vi "Register gRPC Methods.vi"(8 "error in (no error)":errorcluster, 11 "Template Server in":refnum<class "MeasurementService_Template.lvclass">) -> (0 "error out":errorcluster, 3 "Template Server out":refnum<class "MeasurementService_Template.lvclass">)   [LabVIEW 2020, in "LoadRegulation.lvlib" / "MeasurementService_Template.lvclass"]
uses:
  MeasurementService_Template.lvclass
  typeDefs/Server Internal UEs.ctl
  typeDefs/Server Internal Message.ctl
  typeDefs/Server gRPC UEs.ctl
  <vilib>/gRPC/LabVIEW gRPC Library/Server API/typeDefs/gRPCId Cluster.ctl
  <vilib>/gRPC/LabVIEW gRPC Library/Server API/typeDefs/grpcId.ctl
  MeasurementService_Template.lvclass/MeasurementService_Template.ctl
  <vilib>/gRPC/LabVIEW gRPC Library/gprc-lvsupport-release.lvlib
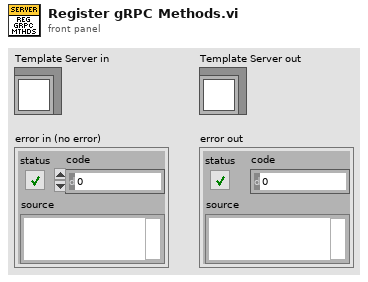
[diagram p1: front panel]
types:
  T1 = typedef "LoadRegulation.lvlib/MeasurementService_Template.lvclass/Server gRPC UEs.ctl" = cluster{"Measurement_v1_MeasurementService_GetMetadata gRPC UE":refnum<user-event>, "Measurement_v1_MeasurementService_Measure gRPC UE":refnum<user-event>, "Measurement_v1_MeasurementService_StopService gRPC UE":refnum<user-event>}
  T2 = typedef "LoadRegulation.lvlib/MeasurementService_Template.lvclass/Server Internal UEs.ctl" = cluster{"Measurement_v1_MeasurementService_GetMetadata Internal UE":refnum<user-event>, "Measurement_v1_MeasurementService_Measure Internal UE":refnum<user-event>, "Measurement_v1_MeasurementService_StopService Internal UE":refnum<user-event>}
  T3 = typedef "gprc-lvsupport-release.lvlib/grpcId.ctl" = u64
  T4 = typedef "LoadRegulation.lvlib/MeasurementService_Template.lvclass/Server Internal Message UE.ctl" = refnum<user-event>
  T5 = typedef "gprc-lvsupport-release.lvlib/gRPCId Cluster UE.ctl" = refnum<user-event>
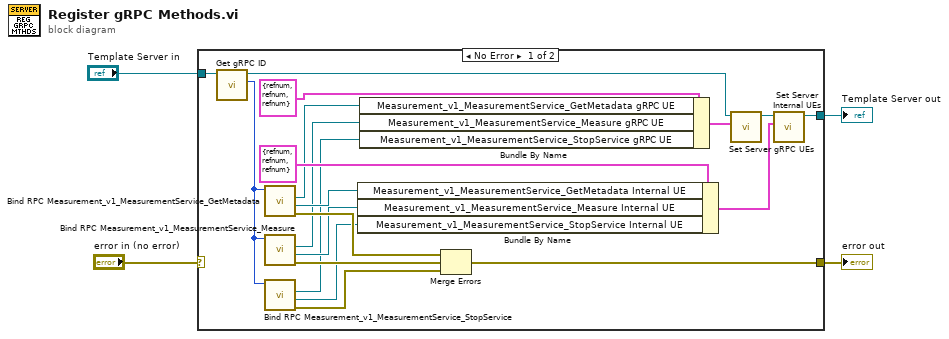
[diagram p0: block diagram]
diagram:
  n1 = case shown="No Error" "error in (no error)" {
    selector: "error in (no error)" -> [_ w24]
    tunnel: "Template Server in" -> [w22 w25]
    tunnel: [w21 w24] -> w3
    tunnel: [w20 w25] -> w2
    frame No Error {
      n2 = call "Get gRPC ID.vi"("OOP Server in"=w22) -> ("gRPC ID"=w14:T3, "OOP Server out"=w23:refnum<class "MeasurementService_Template.lvclass">)  [unwired: 9 in]
      n3 = call "Bind RPC Measurement_v1_MeasurementService_GetMetadata.vi"("gRPCid server in"=w14) -> ("error out"=w13:errorcluster, "Measurement_v1_MeasurementService_GetMetadata Internal UE"=w11:T4, "Measurement_v1_MeasurementService_GetMetadata gRPC UE"=w12:T5)  [unwired: 7 in, 1 out]
      n4 = call "Bind RPC Measurement_v1_MeasurementService_Measure.vi"("gRPCid server in"=w14) -> ("error out"=w10:errorcluster, "Measurement_v1_MeasurementService_Measure Internal UE"=w8:T4, "Measurement_v1_MeasurementService_Measure gRPC UE"=w9:T5)  [unwired: 7 in, 1 out]
      n5 = call "Bind RPC Measurement_v1_MeasurementService_StopService.vi"("gRPCid server in"=w14) -> ("error out"=w7:errorcluster, "Measurement_v1_MeasurementService_StopService Internal UE"=w5:T4, "Measurement_v1_MeasurementService_StopService gRPC UE"=w6:T5)  [unwired: 7 in, 1 out]
      n6 = Bundle By Name ("Bundle Internal UEs")(cluster=T2 {"Measurement_v1_MeasurementService_GetMetadata Internal UE"=refnum, "Measurement_v1_MeasurementService_Measure Internal UE"=refnum, "Measurement_v1_MeasurementService_StopService Internal UE"=refnum} ("Server Internal UEs"), "Measurement_v1_MeasurementService_GetMetadata Internal UE"=w11, "Measurement_v1_MeasurementService_Measure Internal UE"=w8, "Measurement_v1_MeasurementService_StopService Internal UE"=w5) -> (w19:T2)
      n7 = Bundle By Name ("Bundle gRPC UEs")(cluster=T1 {"Measurement_v1_MeasurementService_GetMetadata gRPC UE"=refnum, "Measurement_v1_MeasurementService_Measure gRPC UE"=refnum, "Measurement_v1_MeasurementService_StopService gRPC UE"=refnum} ("gRPC Server Method Events"), "Measurement_v1_MeasurementService_GetMetadata gRPC UE"=w12, "Measurement_v1_MeasurementService_Measure gRPC UE"=w9, "Measurement_v1_MeasurementService_StopService gRPC UE"=w6) -> (w16:T1)
      n8 = Merge Errors(w13, w10, w7) -> (w21:errorcluster)
      n9 = call "Set Server gRPC UEs.vi"("Server RPC Methods"=w16, "OOP Server in"=w23) -> ("OOP Server out"=w17:refnum<class "MeasurementService_Template.lvclass">)  [unwired: 9 in]
      n10 = call "Set Server Internal UEs.vi"("Server Internal UEs"=w19, "OOP Server in"=w17) -> ("OOP Server out"=w20:refnum<class "MeasurementService_Template.lvclass">)  [unwired: 9 in]
    }
    frame Error {
    }
  }
  "error out" <- w3
  "Template Server out" <- w2
